vi "user input.vi"(8 "error in":errorcluster) -> (0 "error out":errorcluster, 3 "Inputs from system":T1)   [LabVIEW 2013, in "user control module.lvclass"]
uses:
  user control module.lvclass
  input user data.ctl
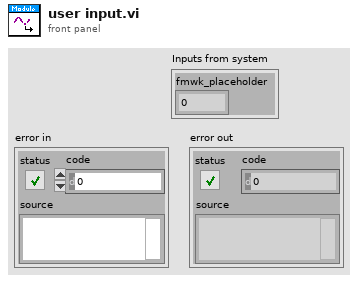
[diagram p1: front panel]
types:
  T1 = typedef "user control module.lvclass/input user data.ctl" = cluster{"fmwk_placeholder":sgl}
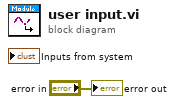
[diagram p0: block diagram]
diagram:
  "error out" <- "error in"
